vi "Add Method to Class from Template.vi"(8 "error in (no error)":errorcluster, 9 "Path to Class":path, 10 "Location of Template":path, 11 "Project in":refnum<vi>) -> (0 "error out":errorcluster, 3 "Project out":refnum<vi>)   [LabVIEW 2016, in "MeasurementMetaData.lvclass"]
doc: "Given a template for a new method, this VI will create a new copy of this VI and add it to a Class. The copy of the new method will be stored in the same locaiton as the .lvclass file"
uses:
  MeasurementMetaData.lvclass
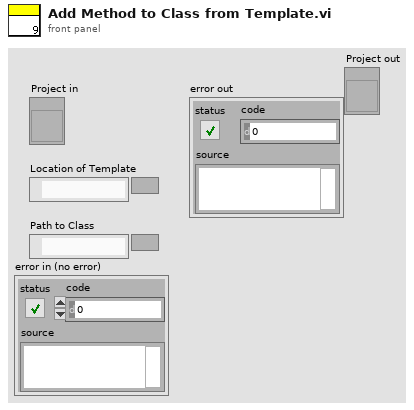
[diagram p1: front panel]
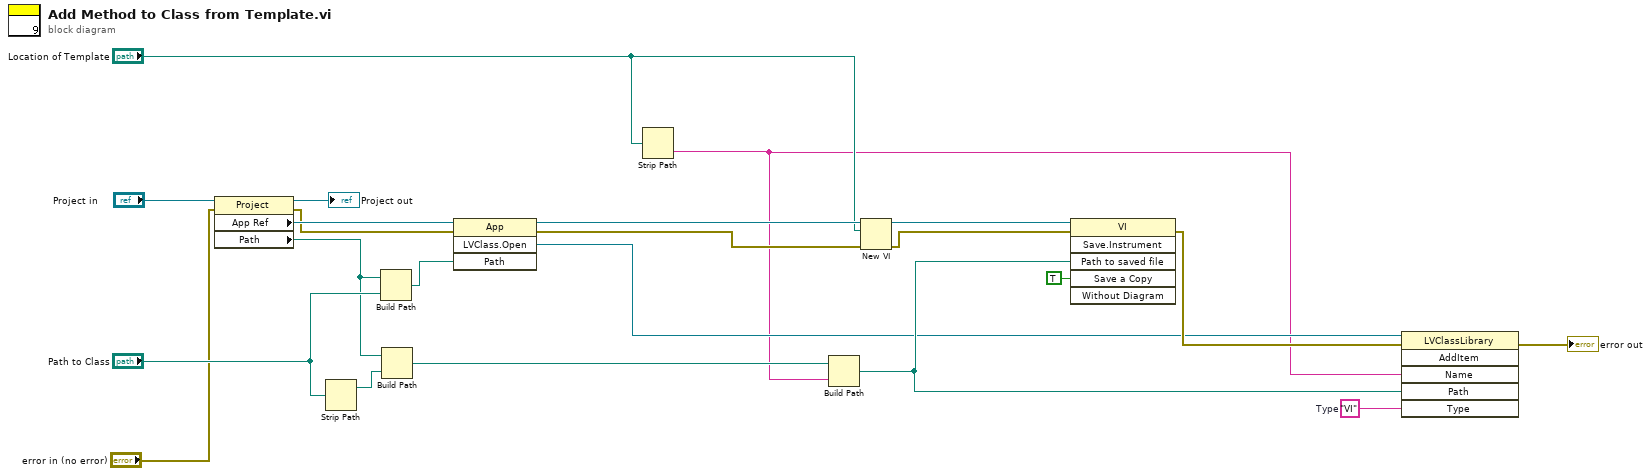
[diagram p0: block diagram]
diagram:
  w11 = "VI"  # Type
  n1 = property class="Project"(reference="Project in", error in="error in (no error)") -> (reference out=→"Project out":refnum<vi>, error out=w1:errorcluster, "App Ref"=w20:refnum<vi>, "Path"=w8:path)
  n2 = Strip Path(path="Path to Class") -> (stripped path=w7:path)  [unwired: 1 out]
  n3 = Build Path(base path=w8, name or relative path="Path to Class") -> (appended path=w22:path)
  n4 = Build Path(base path=w8, name or relative path=w7) -> (appended path=w6:path)
  n5 = invoke class="App" method="LVClass.Open"(reference=w20, error in=w1, "Path"=w22) -> (reference out=w10:refnum<vi>, error out=w18:errorcluster, "LVClass.Open"=w14:refnum<vi>)  [unwired: 1 in, 1 out]
  n6 = Strip Path(path="Location of Template") -> (name=w4:string)  [unwired: 1 out]
  n7 = Build Path(base path=w6, name or relative path=w4) -> (appended path=w15:path)
  n8 = New VI(8:w18, 10:"Location of Template", 11:w10) -> (0:w19:errorcluster, 3:w12:refnum<vi>)  [unwired: 4 in]
  n9 = invoke class="VI" method="Save.Instrument"(reference=w12, error in=w19, "Path to saved file"=w15, "Save a Copy"=TRUE) -> (error out=w16:errorcluster)  [unwired: 2 in, 5 out]
  n10 = invoke class="LVClassLibrary" method="AddItem"(reference=w14, error in=w16, "Name"=w4, "Path"=w15, "Type"=w11) -> (error out=→"error out":errorcluster)  [unwired: 1 in, 5 out]
